vi "AddtoCommand.vi"(6 "Force? (F)":bool, 8 "error in (no error)":errorcluster, 11 "PathTokenizer in":refnum<class "PathTokenizer.lvclass">) -> (0 "error out":errorcluster, 3 "PathTokenizer out":refnum<class "PathTokenizer.lvclass">)   [LabVIEW 2019, in "PathTokenizer.lvclass"]
uses:
  PathTokenizer.lvclass
  PathTokenizer.lvclass/PathTokenizer.ctl
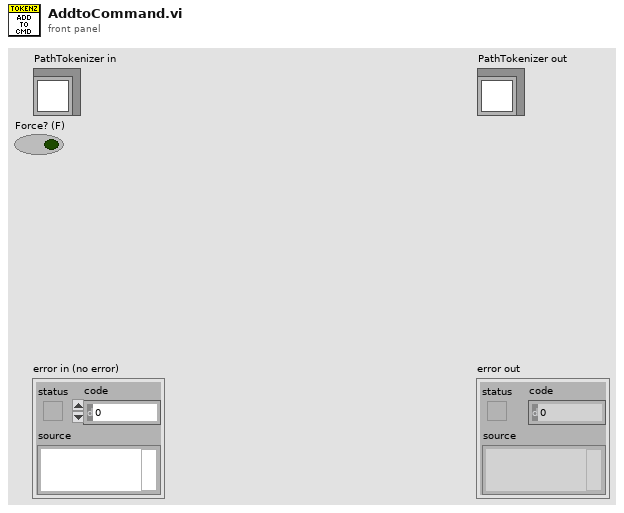
[diagram p1: front panel]
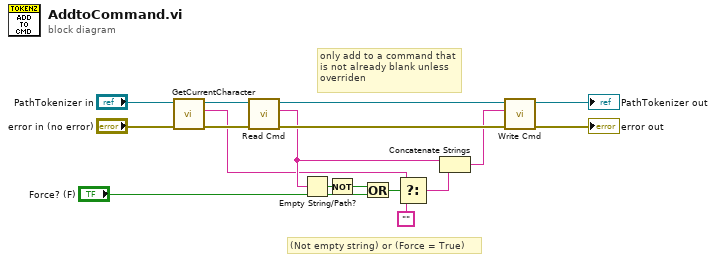
[diagram p0: block diagram]
diagram:
  # "(Not empty string) or (Force = True)"
  # "only add to a command that is not already blank unless overriden"
  n1 = call "GetCurrentCharacter.vi"("error in (no error)"="error in (no error)", "PathTokenizer in"="PathTokenizer in") -> ("error out"=w15:errorcluster, "Current Character"=w2:string, "PathTokenizer out"=w16:refnum<class "PathTokenizer.lvclass">)  [unwired: 7 in]
  n2 = call "Read Cmd.vi"("error in (no error)"=w15, "PathTokenizer in"=w16) -> ("error out"=w12:errorcluster, "Cmd"=w5:string, "PathTokenizer out"=w14:refnum<class "PathTokenizer.lvclass">)  [unwired: 7 in]
  n3 = Empty String/Path?(string/path=w5) -> (empty?=w9:bool)
  n4 = Not(x=w9) -> (.not. x?=w7:bool)
  n5 = Or(x=w7, y="Force? (F)") -> (x .or. y?=w6:bool)
  n6 = Select(t=w2, s=w6, f="" ("Empty String Constant")) -> (s? t:f=w4:string)
  n7 = Concatenate Strings(w5, w4) -> (w3:string)
  n8 = call "Write Cmd.vi"("error in (no error)"=w12, "Cmd"=w3, "PathTokenizer in"=w14) -> ("error out"=→"error out":errorcluster, "PathTokenizer out"=→"PathTokenizer out":refnum<class "PathTokenizer.lvclass">)  [unwired: 7 in]
